vi "Save Settings.vi"(8 "error in (no error)":errorcluster, 11 "IMAQ Display in":refnum<class "HIJ Vision Display.lvclass">) -> (0 "error out":errorcluster, 3 "IMAQ Display out":refnum<class "HIJ Vision Display.lvclass">)   [LabVIEW 2020, in "HIJ Vision Display.lvlib" / "HIJ Vision Display.lvclass"]
uses:
  HIJ Vision Display.lvclass
  HIJ Vision Display.lvclass/HIJ Vision Display.ctl
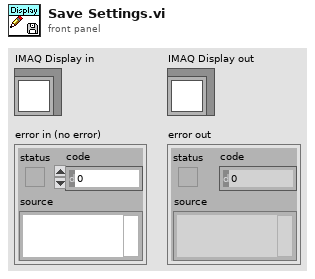
[diagram p1: front panel]
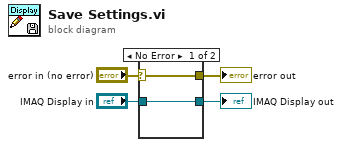
[diagram p0: block diagram]
diagram:
  n1 = case shown="No Error" "error in (no error)" {
    selector: "error in (no error)" -> [w5 w8]
    tunnel: [w5 w8] -> w3
    tunnel: [w6 w7] -> w1
    tunnel: "IMAQ Display in" -> [w6 w7]
    frame No Error {
    }
    frame Error {
    }
  }
  "error out" <- w3
  "IMAQ Display out" <- w1
